vi "Get Server DLL Path.vi"() -> (0 "Server dll path":path)   [LabVIEW 2019, in "Template Client.lvlib" / "gprc-lvsupport.lvlib"]
uses:
  gprc-lvsupport.lvlib
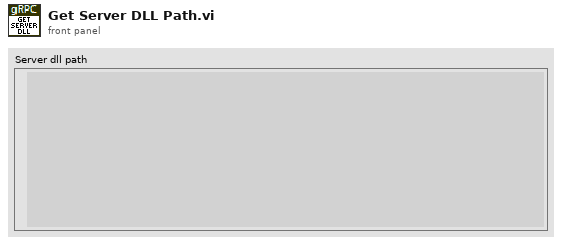
[diagram p1: front panel]
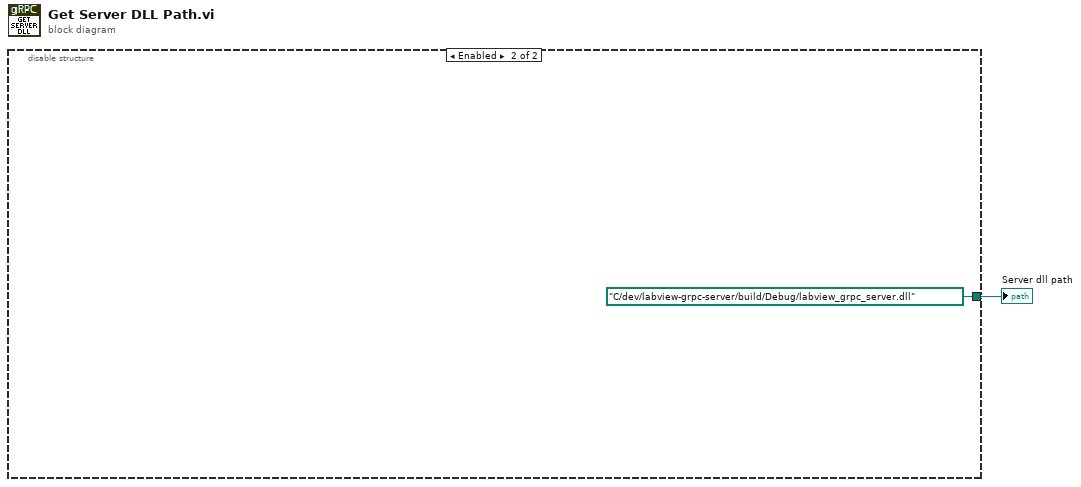
[diagram p0: block diagram]
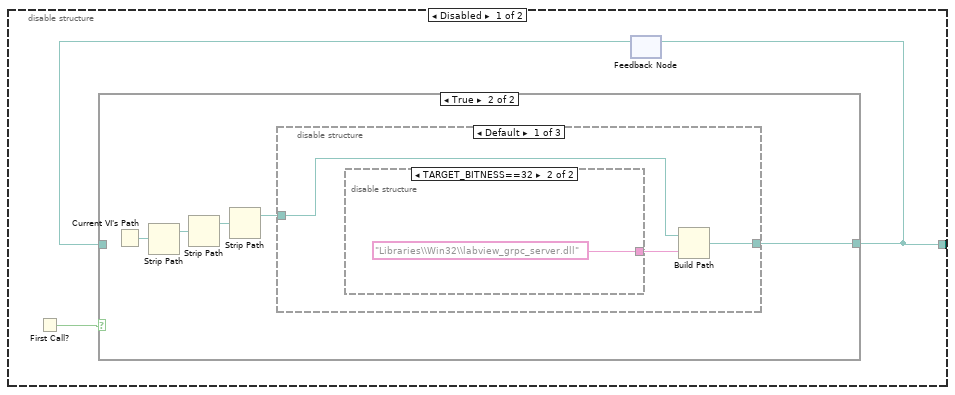
[diagram p2: hidden frame]
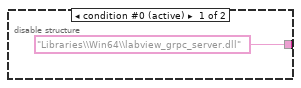
[diagram p4: hidden frame]
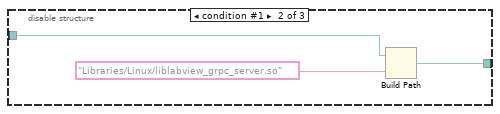
[diagram p5: hidden frame]
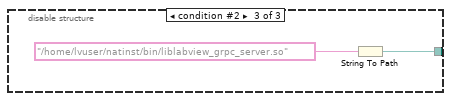
[diagram p6: hidden frame]
diagram:
  n1 = disable-structure shown="Enabled" {
    disable-tunnel: [w3 path "C:/dev/labview-grpc-server/build/Debug/labview_grpc_server.dll" ("Server dll path")] -> w1
    frame Disabled {
      n2 = First Call?() -> (First Call?: T/F=w4:bool)
      n3 = feedback #1() -> (w2:path)  [unwired: 1 in]
      n4 = case shown="True" w4 {
        tunnel: [w5 w6] -> w3
        tunnel: w2 -> [w5 _]
        frame False {
        }
        frame True {
          n5 = Current VI's Path() -> (path=w9:path)
          n6 = Strip Path(path=w9) -> (stripped path=w10:path)  [unwired: 1 out]
          n7 = Strip Path(path=w10) -> (stripped path=w8:path)  [unwired: 1 out]
          n8 = Strip Path(path=w8) -> (stripped path=w7:path)  [unwired: 1 out]
          n9 = disable-structure shown="Default" {
            disable-tunnel: w7 -> [w12 w18 _]
            disable-tunnel: [w11 w17 w19] -> w6
            frame condition #0 (active) {
              n10 = disable-structure shown="TARGET_BITNESS==32" {
                disable-tunnel: ["Libraries\\Win64\\labview_grpc_server.dll" ("name or relative path") "Libraries\\Win32\\labview_grpc_server.dll" ("name or relative path")] -> w13
                frame condition #0 (active) {
                }
                frame condition #1 {
                }
              }
              n11 = Build Path(base path=w12, name or relative path=w13) -> (appended path=w11:path)
            }
            frame condition #1 {
              n12 = Build Path(base path=w18, name or relative path="Libraries/Linux/liblabview_grpc_server.so") -> (appended path=w17:path)
            }
            frame condition #2 {
              n13 = String To Path(string="/home/lvuser/natinst/bin/liblabview_grpc_server.so" ("name or relative path")) -> (path=w19:path)
            }
          }
        }
      }
      n14 = feedback-in #1(w3) -> ()
    }
    frame Enabled {
    }
  }
  "Server dll path" <- w1
